vi "Teardown Camera.vi"(4 "error in (no error)":errorcluster) -> (0 "error out":errorcluster, 3 "function return":i32)   [LabVIEW 2020, in "ThorConfocal.lvlib"]
doc: "long TeardownCamera();"
uses:
  ThorConfocal.lvlib
  ThorConfocal.dll
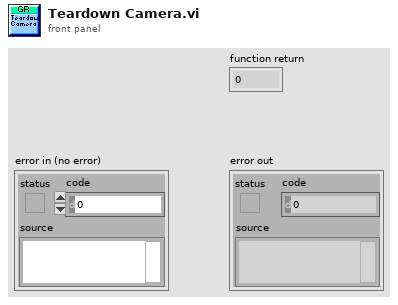
[diagram p1: front panel]
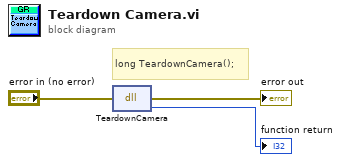
[diagram p0: block diagram]
diagram:
  # "long TeardownCamera();"
  n1 = dll-call lib="D:/software/TweezerTron/ThorConfocal.dll" fn="TeardownCamera"(error in="error in (no error)") -> (error out=→"error out":errorcluster, "return type"=→"function return":i32)  [unwired: 2 in, 1 out]
